vi "Joystick corrector.vi"(8 "rate":dbl, 10 "Joystick":dbl) -> (2 "output":dbl)   [LabVIEW 2017]
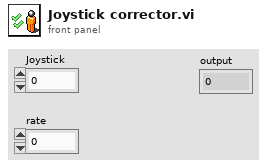
[diagram p1: front panel]
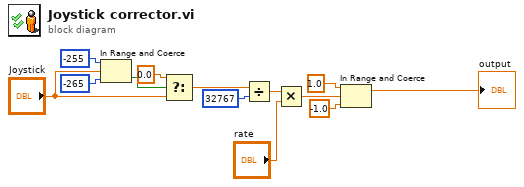
[diagram p0: block diagram]
diagram:
  n1 = In Range and Coerce(upper limit=-255, x="Joystick", lower limit=-265) -> (In Range?=w13:bool)  [unwired: 1 out]
  n2 = Select(t=0.0, s=w13, f="Joystick") -> (s? t:f=w11:dbl)
  n3 = Divide(x=w11, y=32767) -> (x/y=w6:dbl)
  n4 = Multiply(x=w6, y="rate") -> (x*y=w2:dbl)
  n5 = In Range and Coerce(upper limit=1.0, x=w2, lower limit=-1.0) -> (coerced(x)=→"output":dbl)  [unwired: 1 out]
